vi "Create Write Endpoint.vi"(7 "Refs":T1, 8 "error in (no error)":errorcluster, 10 "Type Descriptor":T2, 11 "Channel Term":refnum<vi>) -> (0 "error out":errorcluster, 3 "Element Term":refnum<vi>)   [LabVIEW 2022 SP3, in "FlexBlocks Support.lvlib"]
uses:
  FlexBlocks Support.lvlib
  Type Descriptor.ctl
  Terminal Direction.ctl
  Value Mode.ctl
  Special Terminal.ctl
  SM Refs.ctl
  <vilib>/Utility/miscctls.llb/LVPointTypeDef.ctl
  Status Terminals.ctl
  Write Terminals.ctl
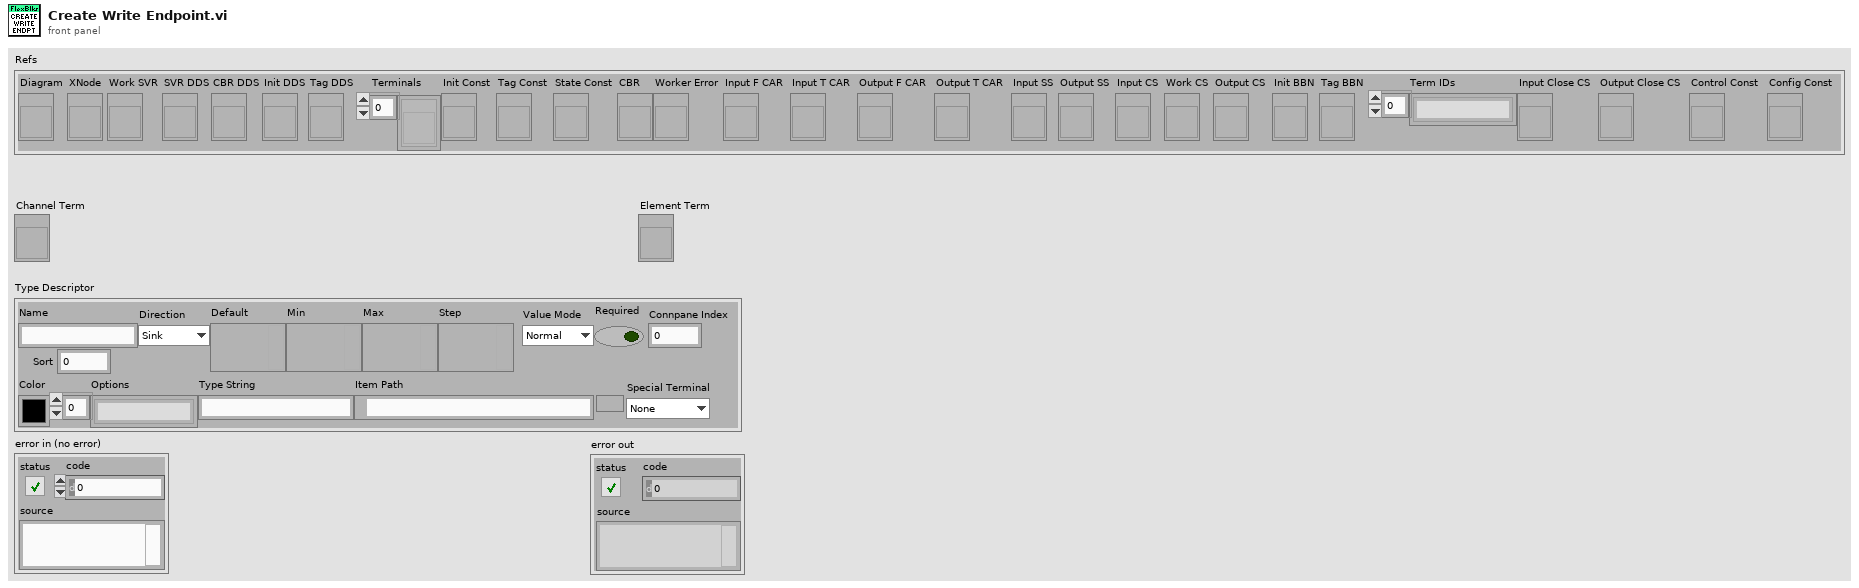
[diagram p1: front panel]
types:
  T1 = typedef "FlexBlocks Support.lvlib/SM Refs.ctl" = cluster{"Diagram":refnum<vi>, "XNode":refnum<vi>, "Work SVR":refnum<vi>, "SVR DDS":refnum<vi>, "CBR DDS":refnum<vi>, "Init DDS":refnum<vi>, "Tag DDS":refnum<vi>, "Terminals":refnum<vi>[], "Init Const":refnum<vi>, "Tag Const":refnum<vi>, "State Const":refnum<vi>, "CBR":refnum<vi>, "Worker Error":refnum<vi>, "Input F CAR":refnum<vi>, "Input T CAR":refnum<vi>, "Output F CAR":refnum<vi>, "Output T CAR":refnum<vi>, "Input SS":refnum<vi>, "Output SS":refnum<vi>, "Input CS":refnum<vi>, "Work CS":refnum<vi>, "Output CS":refnum<vi>, "Init BBN":refnum<vi>, "Tag BBN":refnum<vi>, "Term IDs":string[], "Input Close CS":refnum<vi>, "Output Close CS":refnum<vi>, "Control Const":refnum<vi>, "Config Const":refnum<vi>}
  T2 = typedef "FlexBlocks Support.lvlib/Type Descriptor.ctl" = cluster{"Name":string, "Direction":T3, "Default":variant, "Min":variant, "Max":variant, "Step":variant, "Value Mode":T4, "Color":u32, "Options":string[], "Type String":string, "Item Path":path, "Required":bool, "Connpane Index":i32, "Special Terminal":T5, "Sort":i32}
  T3 = typedef "FlexBlocks Support.lvlib/Terminal Direction.ctl" = enum16{"Sink", "Source"}
  T4 = typedef "FlexBlocks Support.lvlib/Value Mode.ctl" = enum16{"Normal", "Range", "Select"}
  T5 = typedef "FlexBlocks Support.lvlib/Special Terminal.ctl" = enum16{"None", "Action", "Init", "Tag", "State in", "State out", "Error", "Control", "Config"}
  T6 = typedef "FlexBlocks Support.lvlib/Write Terminals.ctl" = enum16{"Timeout mS", "Synchronous", "Element", "Close", "NC 4", "NC 5", "Timed Out", "FlexChannel", "NC 8", "Closed"}
  T7 = typedef "FlexBlocks Support.lvlib/Status Terminals.ctl" = enum16{"# Pending Write", "# Pending Read", "Usage Ratio", "Queued Count", "Closed?", "Updated", "NC 6", "Sequence", "NC 8", "NC 9", "NC 10", "FlexChannel"}
  T8 = typedef "LVPointTypeDef.ctl" = cluster{"Horizontal":i16, "Vertical":i16}
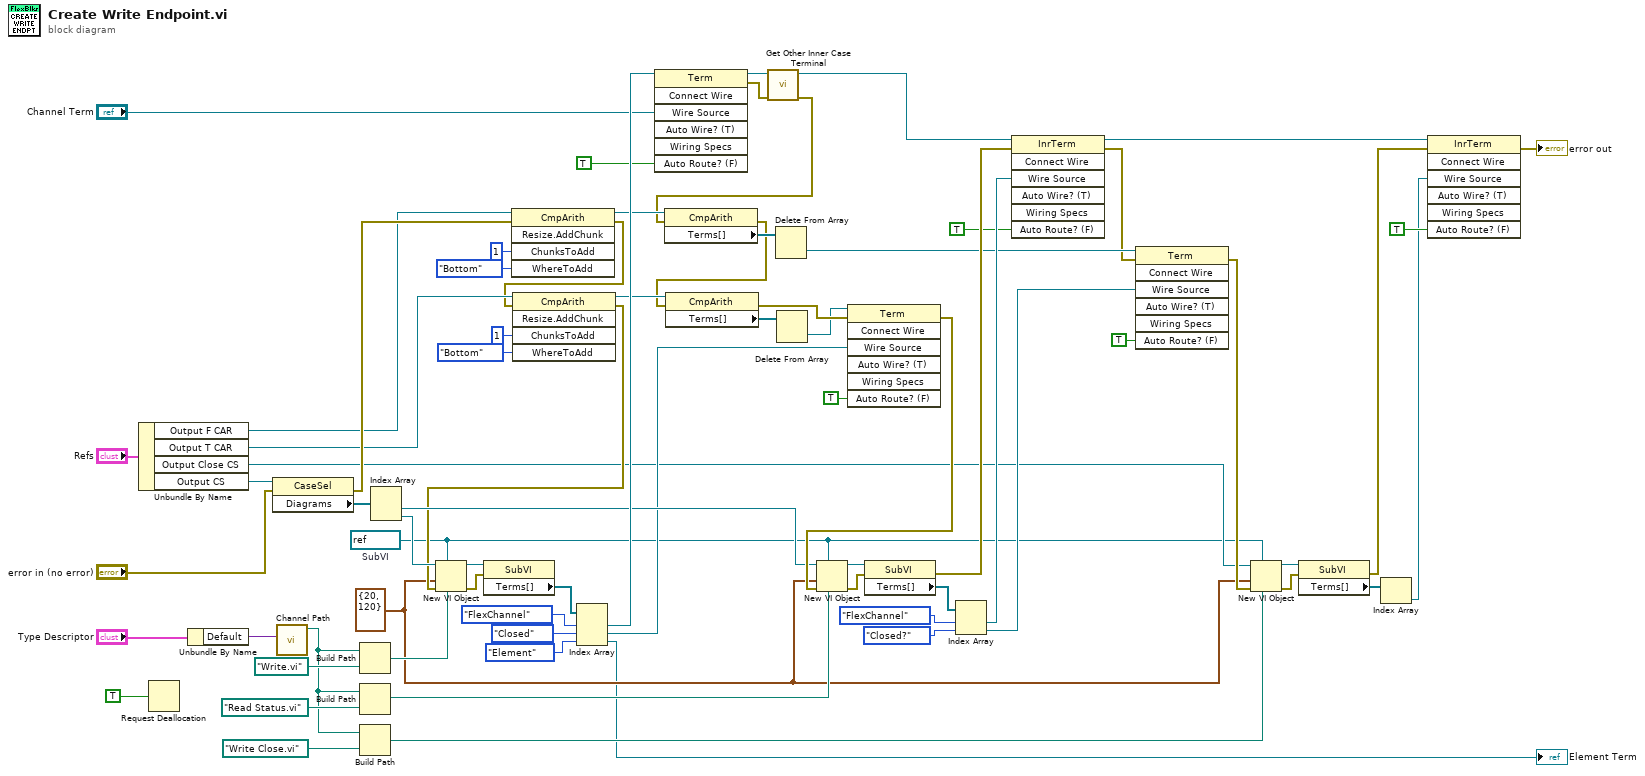
[diagram p0: block diagram]
diagram:
  w4 = T8 {"Horizontal"=20, "Vertical"=120} ("location")
  w2 = refnum<vi> refnum  # SubVI
  n1 = Unbundle By Name("Refs") -> ("Output F CAR"=w35:refnum<vi>, "Output T CAR"=w45:refnum<vi>, "Output Close CS"=w3:refnum<vi>, "Output CS"=w58:refnum<vi>)
  n2 = Request Deallocation(TRUE ("flag")) -> ()
  n3 = Unbundle By Name("Type Descriptor") -> ("Default"=w69:variant)
  n4 = property class="CaseSel"(reference=w58, error in="error in (no error)") -> (error out=w73:errorcluster, "Diagrams"=w57:refnum<vi>[])  [unwired: 1 out]
  n5 = call "Channel Path.vi"("Variant"=w69) -> ("Channel Folder Path"=w15:path)  [unwired: 9 in, 1 out]
  n6 = Build Path(base path=w15, name or relative path=path "Write.vi") -> (appended path=w65:path)
  n7 = Build Path(base path=w15, name or relative path=path "Read Status.vi") -> (appended path=w53:path)
  n8 = Build Path(base path=w15, name or relative path=path "Write Close.vi") -> (appended path=w5:path)
  n9 = Index Array(array=w57) -> (element #1=w42:refnum<vi>, element #2=w56:refnum<vi>)  [unwired: 2 in]
  n10 = invoke class="CmpArith" method="Resize.AddChunk"(reference=w35, error in=w73, "ChunksToAdd"=u8 1 ("Chunks To Add"), "WhereToAdd"=enum8{"Bottom", "Top"}."Bottom" ("Where To Add")) -> (reference out=w34:refnum<vi>, error out=w23:errorcluster)  [unwired: 1 in, 3 out]
  n11 = invoke class="CmpArith" method="Resize.AddChunk"(reference=w45, error in=w23, "ChunksToAdd"=u8 1 ("Chunks To Add"), "WhereToAdd"=enum8{"Bottom", "Top"}."Bottom" ("Where To Add")) -> (reference out=w41:refnum<vi>, error out=w22:errorcluster)  [unwired: 1 in, 3 out]
  n12 = New VI Object(vi object class=w2, owner refnum=w56, position/next to=w4, 6:w65, 8:w22) -> (object refnum=w64:refnum<vi>, 0:w63:errorcluster)  [unwired: 3 in]
  n13 = property class="SubVI"(reference=w64, error in=w63) -> ("Terms[]"=w62:refnum<vi>[])  [unwired: 2 out]
  n14 = Index Array(array=w62, index #1=Write_Terminals."FlexChannel" ("Write Terminals"), index #2=Write_Terminals."Closed" ("Write Terminals"), index #3=Write_Terminals."Element" ("Write Terminals")) -> (element #1=w61:refnum<vi>, element #2=w17:refnum<vi>, element #3=→"Element Term":refnum<vi>)
  n15 = invoke class="Term" method="Connect Wire"(reference=w61, "Wire Source"="Channel Term", "Auto Route? (F)"=TRUE) -> (reference out=w51:refnum<vi>, error out=w50:errorcluster)  [unwired: 4 in, 5 out]
  n16 = call "Get Other Inner Case Terminal.vi"("error in (no error)"=w50, "Term"=w51) -> ("error out"=w27:errorcluster, "Other InnerTerm"=w47:refnum<vi>)  [unwired: 8 in]
  n17 = property class="CmpArith"(reference=w34, error in=w27) -> (error out=w26:errorcluster, "Terms[]"=w38:refnum<vi>[])  [unwired: 1 out]
  n18 = property class="CmpArith"(reference=w41, error in=w26) -> (error out=w25:errorcluster, "Terms[]"=w40:refnum<vi>[])  [unwired: 1 out]
  n19 = Delete From Array(array=w38) -> (deleted portion=w31:refnum<vi>)  [unwired: 2 in, 1 out]
  n20 = Delete From Array(array=w40) -> (deleted portion=w18:refnum<vi>)  [unwired: 2 in, 1 out]
  n21 = invoke class="Term" method="Connect Wire"(reference=w18, error in=w25, "Wire Source"=w17, "Auto Route? (F)"=TRUE) -> (error out=w72:errorcluster)  [unwired: 3 in, 6 out]
  n22 = New VI Object(vi object class=w2, owner refnum=w42, position/next to=w4, 6:w53, 8:w72) -> (object refnum=w54:refnum<vi>, 0:w55:errorcluster)  [unwired: 3 in]
  n23 = property class="SubVI"(reference=w54, error in=w55) -> (error out=w33:errorcluster, "Terms[]"=w52:refnum<vi>[])  [unwired: 1 out]
  n24 = Index Array(array=w52, index #1=Status_Terminals."FlexChannel" ("Status Terminals"), index #2=Status_Terminals."Closed?" ("Status Terminals")) -> (element #1=w46:refnum<vi>, element #2=w28:refnum<vi>)
  n25 = invoke class="InrTerm" method="Connect Wire"(reference=w47, error in=w33, "Wire Source"=w46, "Auto Route? (F)"=TRUE) -> (reference out=w8:refnum<vi>, error out=w30:errorcluster)  [unwired: 3 in, 5 out]
  n26 = invoke class="Term" method="Connect Wire"(reference=w31, error in=w30, "Wire Source"=w28, "Auto Route? (F)"=TRUE) -> (error out=w12:errorcluster)  [unwired: 3 in, 6 out]
  n27 = New VI Object(vi object class=w2, owner refnum=w3, position/next to=w4, 6:w5, 8:w12) -> (object refnum=w14:refnum<vi>, 0:w13:errorcluster)  [unwired: 3 in]
  n28 = property class="SubVI"(reference=w14, error in=w13) -> (error out=w7:errorcluster, "Terms[]"=w10:refnum<vi>[])  [unwired: 1 out]
  n29 = Index Array(array=w10) -> (element=w9:refnum<vi>)  [unwired: 1 in]
  n30 = invoke class="InrTerm" method="Connect Wire"(reference=w8, error in=w7, "Wire Source"=w9, "Auto Route? (F)"=TRUE) -> (error out=→"error out":errorcluster)  [unwired: 3 in, 6 out]
